vi "Add Entry - Directory.vi"(7 "Directory":string[](array[string]), 8 "error in (no error)":errorcluster, 9 "Value":variant, 10 "Key":string caption="Name", 11 "Registry in":refnum<class "Registry.lvclass">) -> (0 "error out":errorcluster, 2 "Replaced?":bool, 3 "Registry out":refnum<class "Registry.lvclass">)   [LabVIEW 2020, in "BCI-1553 API.lvlib" / "Registry.lvlib" / "Registry.lvclass"]
uses:
  Registry.lvclass
  Registry.lvclass/Registry.ctl
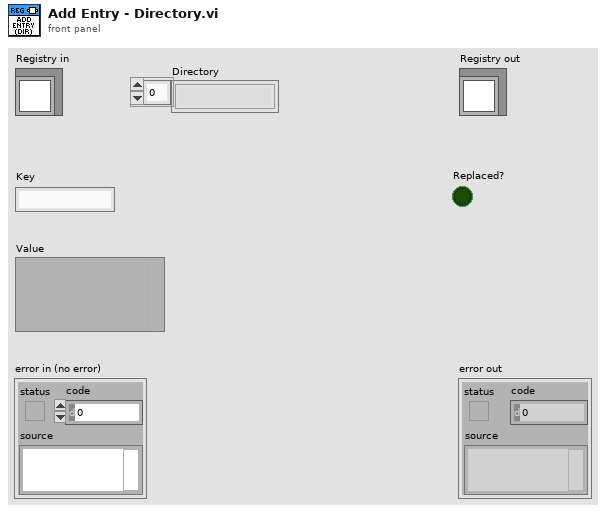
[diagram p1: front panel]
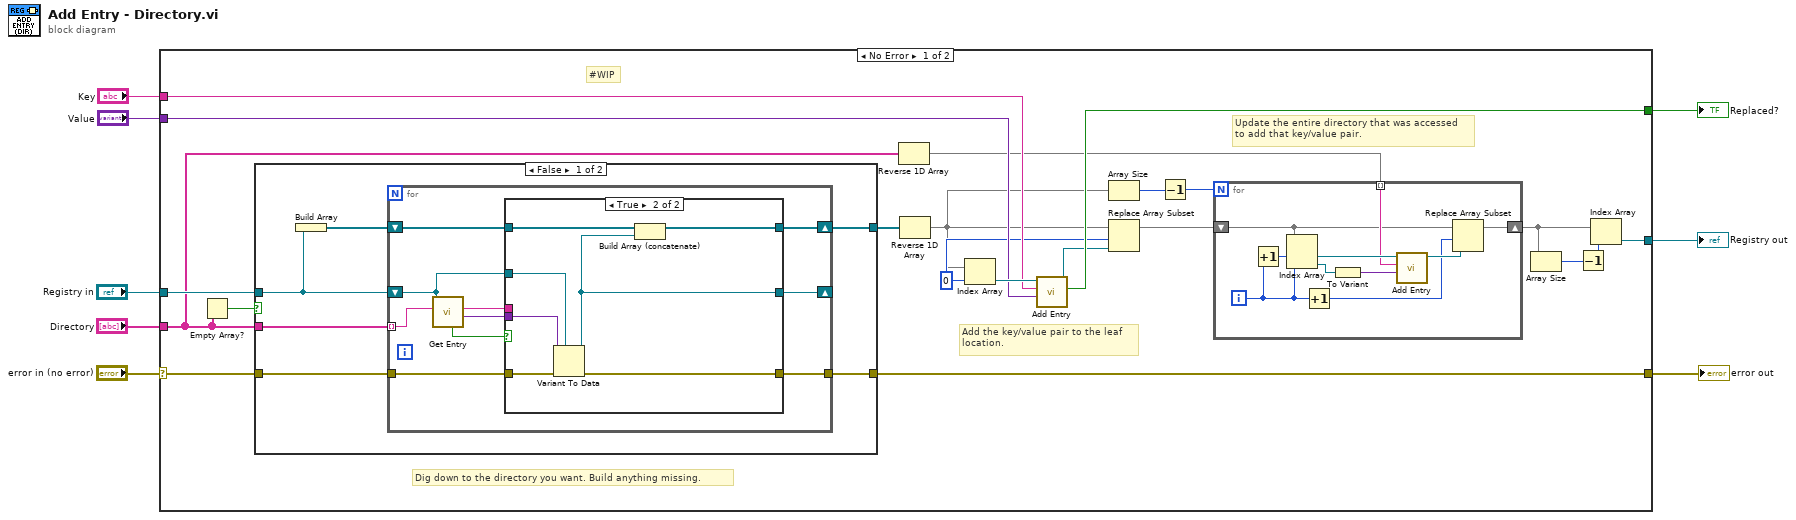
[diagram p0: block diagram]
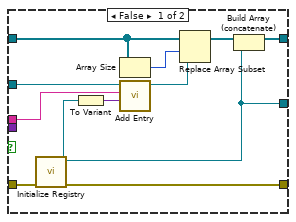
[diagram p2: hidden frame]
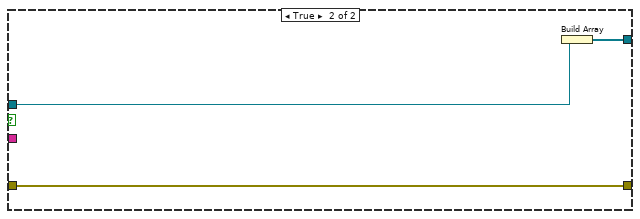
[diagram p3: hidden frame]
diagram:
  n1 = case shown="No Error" "error in (no error)" {
    selector: "error in (no error)" -> [w28 w78]
    tunnel: [w9 w78] -> w6
    tunnel: "Registry in" -> [w29 w77]
    tunnel: "Directory" -> [w15 _]
    tunnel: [w10 w77] -> w2
    tunnel: "Key" -> [w24 _]
    tunnel: "Value" -> [w23 _]
    tunnel: [w22 _] -> w1
    frame No Error {
      w19 = 0
      # "Update the entire directory that was accessed\nto add that key/value pair."
      # "Add the key/value pair to the leaf\nlocation."
      # "Dig down to the directory you want. Build anything missing."
      # "#WIP"
      n2 = Empty Array?(array=w15) -> (empty?=w27:bool)
      n3 = case shown="False" w27 {
        tunnel: w29 -> [w41 w75]
        tunnel: w15 -> [w45 _]
        tunnel: w28 -> [w44 w76]
        tunnel: [w43 w76] -> w9
        tunnel: [w42 w74] -> w26
        frame False {
          n4 = Build Array(w41) -> (w40:refnum<class "Registry.lvclass">[])
          n5 = for {
            tunnel: w45 -> [w55] mode=indexing
            tunnel: w44 -> [w49]
            tunnel: [w48] -> w43
            shift-right: [w50] -> _
            shift-left: w41 -> [w51]
            shift-right: [w46] -> w42
            shift-left: w40 -> [w47]
            n6 = call "Get Entry.vi"("Key"=w55, "Registry in"=w51) -> ("Value"=w54:variant, "Key Out"=w52:string, "Found?"=w53:bool)  [unwired: 6 in, 1 out]
            n7 = case shown="True" w53 {
              tunnel: w51 -> [w66 w73]
              tunnel: w54 -> [_ w72]
              tunnel: [w60 w68] -> w50
              tunnel: w49 -> [w63 w71]
              tunnel: [w62 w70] -> w48
              tunnel: w52 -> [w65 _]
              tunnel: w47 -> [w59 w69]
              tunnel: [w61 w67] -> w46
              frame False {
                n8 = call "Initialize Registry.vi"("error in (no error)"=w63) -> ("error out"=w62:errorcluster, "Registry out"=w60:refnum<class "Registry.lvclass">)  [unwired: 9 in]
                n9 = To Variant(anything=w60) -> (Variant=w64:variant)
                n10 = Array Size(array=w59) -> (size(s)=w57:i32)
                n11 = call "Add Entry.vi"("Value"=w64, "Key"=w65, "Registry in"=w66) -> ("Registry out"=w56:refnum<class "Registry.lvclass">)  [unwired: 6 in, 2 out]
                n12 = Replace Array Subset(array=w59, new element=w56, index=w57) -> (w58:refnum<class "Registry.lvclass">[])
                n13 = Build Array (concatenate)(w58, w60) -> (w61:refnum<class "Registry.lvclass">[])
              }
              frame True {
                n14 = Variant To Data(error in=w71, type=w73, Variant=w72) -> (data=w68:refnum<class "Registry.lvclass">, error out=w70:errorcluster)
                n15 = Build Array (concatenate)(w69, w68) -> (w67:refnum<class "Registry.lvclass">[])
              }
            }
          }
        }
        frame True {
          n16 = Build Array(w75) -> (w74:refnum<class "Registry.lvclass">[])
        }
      }
      n17 = Reverse 1D Array(array=w15) -> (reversed array=w14:string[])
      n18 = Reverse 1D Array(array=w26) -> (reversed array=w18:refnum<class "Registry.lvclass">[])
      n19 = Index Array(array=w18, index=w19) -> (element=w25:refnum<class "Registry.lvclass">)
      n20 = call "Add Entry.vi"("Value"=w23, "Key"=w24, "Registry in"=w25) -> ("Replaced?"=w22:bool, "Registry out"=w20:refnum<class "Registry.lvclass">)  [unwired: 6 in, 1 out]
      n21 = Array Size(array=w18) -> (size(s)=w17:i32)
      n22 = Replace Array Subset(array=w18, new element=w20, index=w19) -> (w21:refnum<class "Registry.lvclass">[])
      n23 = Decrement(x=w17) -> (x-1=w16:i32)
      n24 = for {
        N: w16 -> [_]
        shift-right: [w30] -> w11
        shift-left: w21 -> [w34]
        tunnel: w14 -> [w35] mode=indexing
        i -> [w32]
        n25 = Increment(x=w32) -> (x+1=w39:i32)
        n26 = Index Array(array=w34, index #1=w39, index #2=w32) -> (element #1=w37:refnum<class "Registry.lvclass">, element #2=w38:refnum<class "Registry.lvclass">)
        n27 = Increment(x=w32) -> (x+1=w31:i32)
        n28 = To Variant(anything=w38) -> (Variant=w36:variant)
        n29 = call "Add Entry.vi"("Value"=w36, "Key"=w35, "Registry in"=w37) -> ("Registry out"=w33:refnum<class "Registry.lvclass">)  [unwired: 6 in, 2 out]
        n30 = Replace Array Subset(array=w34, new element=w33, index=w31) -> (w30:refnum<class "Registry.lvclass">[])
      }
      n31 = Array Size(array=w11) -> (size(s)=w13:i32)
      n32 = Decrement(x=w13) -> (x-1=w12:i32)
      n33 = Index Array(array=w11, index=w12) -> (element=w10:refnum<class "Registry.lvclass">)
    }
    frame Error {
    }
  }
  "error out" <- w6
  "Registry out" <- w2
  "Replaced?" <- w1
